vi "Read_Earlier_Channels.vi"(0 "Present scan array":dbl[](array[numeric]) format="%.2f", 2 "Ch names":string[](array[string]), 3 "Desired Channels":string[](array[string])) -> (1 "Scan comments":string, 5 "Index 0":dbl format="%.2f", 6 "Index 1":dbl format="%.2f", 7 "Index 2":dbl format="%.2f", 8 "Index 3":dbl format="%.2f")   [LabVIEW 2010]
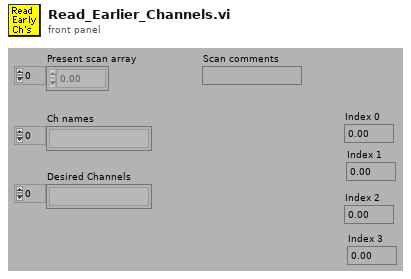
[diagram p1: front panel]
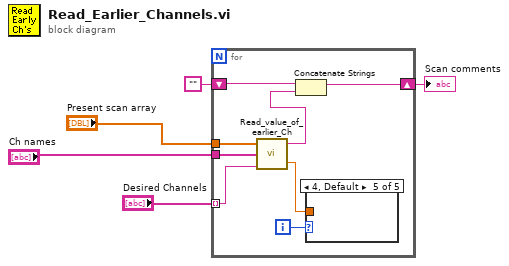
[diagram p0: block diagram]
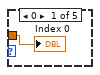
[diagram p2: hidden frame]
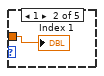
[diagram p3: hidden frame]
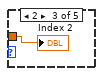
[diagram p4: hidden frame]
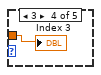
[diagram p5: hidden frame]
diagram:
  n1 = for {
    tunnel: "Present scan array" -> [w13]
    tunnel: "Ch names" -> [w12]
    tunnel: "Desired Channels" -> [w11] mode=indexing
    shift-right: [w8] -> w5
    shift-left: "" -> [w10]
    i -> [w7]
    n2 = call "Read_value_of_earlier_Ch.vi"("Desired Ch to Read"=w11, "Ch names"=w12, "Present scan array"=w13) -> ("Value"=w6:dbl, "Scan comment"=w9:string)  [unwired: 1 in]
    n3 = Concatenate Strings(w10, w9) -> (w8:string)
    n4 = case shown="4, Default" w7 {
      tunnel: w6 -> [w14 w15 w16 w17 _]
      frame 0 {
        "Index 0" <- w14
      }
      frame 1 {
        "Index 1" <- w15
      }
      frame 2 {
        "Index 2" <- w16
      }
      frame 3 {
        "Index 3" <- w17
      }
      frame 4, Default {
      }
    }
  }
  "Scan comments" <- w5
